vi "Begin.vi"(11 "Image Size":T1=enum."160x120") -> (0 "error out":errorcluster)   [LabVIEW 2012]
doc: "Called before other user functions, this VI is expected to open initial I/O refnums, load in file data, and do all program initialization. Notice that the <B>error out</B> terminal is simply used for data flow. Wiring it to other structures or subVIs ensures that this VI runs first."
uses:
  <vilib>/Rock Robotics/WPI/Camera/WPI_CameraImageSize.ctl
  <vilib>/Rock Robotics/WPI/Camera/WPI_CameraWhite Balance Values.ctl
  <vilib>/Rock Robotics/WPI/Camera/WPI_CameraExposure Values.ctl
  <vilib>/Rock Robotics/WPI/Camera/WPI_CameraFrameRate.ctl
  <vilib>/Rock Robotics/WPI/DriverStation/WPI_DriverStationRobotMode2.ctl
  <vilib>/Rock Robotics/SystemInterfaces/DIO/FPGA_DIOChannel.ctl
  <vilib>/Rock Robotics/SystemInterfaces/AI/FPGA_AIGyroChannel.ctl
  <vilib>/Rock Robotics/WPI/Relay/WPI_RelayDirection.ctl
  <vilib>/Rock Robotics/SystemInterfaces/DIO/FPGA_DIORelayChannel.ctl
  <vilib>/Rock Robotics/SystemInterfaces/AI/FPGA_AIChannel.ctl
  <vilib>/Rock Robotics/SystemInterfaces/DIO/FPGA_DIOPWMChannel.ctl
  <vilib>/Rock Robotics/WPI/Joystick/WPI_JoystickDeviceEnum.ctl
  <vilib>/Rock Robotics/SystemInterfaces/Typedef/FPGA_TypedefDigitalModule.ctl
  Robot Global Data.vi
  <vilib>/Rock Robotics/WPI/MotorControl/WPI_MotorControlOpen Victor.vi
  <vilib>/Rock Robotics/WPI/MotorControl/WPI_MotorControlOpen Jaguar.vi
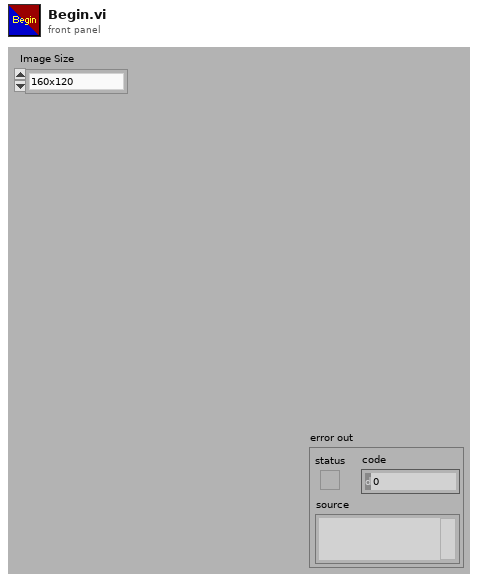
[diagram p1: front panel]
types:
  T1 = typedef "WPI_CameraImageSize.ctl" = enum16{"640x480", "320x240", "160x120"}
  T2 = typedef "FPGA_DIOChannel.ctl" = enum8{"DIO 1", "DIO 2", "DIO 3", "DIO 4", "DIO 5", "DIO 6", "DIO 7", "DIO 8", "DIO 9", "DIO 10", "DIO 11", "DIO 12", "DIO 13", "DIO 14", "Invalid"}
  T3 = typedef "FPGA_TypedefDigitalModule.ctl" = enum16{"Digital Module 1", "Digital Module 2"}
  T4 = typedef "WPI_JoystickDeviceEnum.ctl" = enum16{"USB 1", "USB 2", "USB 3", "USB 4", "Kinect 1", "Kinect 2"}
  T5 = typedef "FPGA_DIOPWMChannel.ctl" = enum8{"PWM 1", "PWM 2", "PWM 3", "PWM 4", "PWM 5", "PWM 6", "PWM 7", "PWM 8", "PWM 9", "PWM 10", "Invalid"}
  T6 = typedef "FPGA_AIChannel.ctl" = enum8{"AI 1", "AI 2", "AI 3", "AI 4", "AI 5", "AI 6", "AI 7", "AI 8", "Invalid"}
  T7 = typedef "FPGA_DIORelayChannel.ctl" = enum8{"Relay 1", "Relay 2", "Relay 3", "Relay 4", "Relay 5", "Relay 6", "Relay 7", "Relay 8", "Invalid"}
  T8 = typedef "WPI_RelayDirection.ctl" = enum16{"Both directions", "Forward only", "Reverse only"}
  T9 = typedef "FPGA_AIGyroChannel.ctl" = enum8{"AI 1", "AI 2", "Invalid"}
  T10 = typedef "WPI_DriverStationRobotMode2.ctl" = enum16{"Autonomous Disabled", "Autonomous Enabled", "Teleop Disabled", "Teleop Enabled", "Timeout", "Finish", "Test Disabled", "Test Enabled"}
  T11 = typedef "WPI_CameraFrameRate.ctl" = u32
  T12 = typedef "WPI_CameraExposure Values.ctl" = enum16{"Auto", "Flicker-free 50 Hz", "Flicker-free 60 Hz", "Hold current"}
  T13 = typedef "WPI_CameraWhite Balance Values.ctl" = enum16{"Auto", "Fixed indoor", "Fixed outdoor 1", "Fixed outdoor 2", "Fixed fluorescent 1", "Fixed fluorescent 2", "Hold current"}
  T14 = typedef "WPI_DigitalInputDevRef.ctl" = cluster{"DevStatus":errorcluster, "DIO Channel":T2, "Digital Module":T3}
  T15 = typedef "WPI_MotorControlDeviceRef.ctl" = cluster{"DeviceStatus":errorcluster, "Type":enum16{"PWM", "CAN"}, "PWM":cluster{"Digital Module":T3, "PWM Channel":T5, "DeadBand":T16}, "CAN":cluster{"Device Number":u8, "Control Mode":T17, "Semaphore":T18, "Max Vout":dbl}, "Invert":bool, "TransformRef":T19, "InvTransformRef":T19}
  T16 = typedef "WPI_PWMDeadband.ctl" = cluster{"Name":string, "maxPositivePwm":i32, "minPositivePwm":i32, "centerPwm":i32, "maxNegativePwm":i32, "minNegativePwm":i32, "angularRange":u16}
  T17 = typedef "WPI_CANJaguar_ControlMode.ctl" = enum8{"Percent VBus", "Current", "Speed", "Position", "Voltage"}
  T18 = typedef "Semaphore RefNum" = refnum<k1>
  T19 = typedef "WPI_PWMTransform_ConPane.ctl" = refnum<vi>
  T20 = typedef "WPI_ServoDeviceRef.ctl" = cluster{"DeviceStatus":errorcluster, "Digital Module":T3, "PWM Channel":T5, "DeadBand":T16}
  T21 = typedef "WPI_RelayDevRef.ctl" = cluster{"DevStatus":errorcluster, "Relay Channel":T7, "Digital Module":T3, "Relay Direction":T8}
  T22 = typedef "WPI_AnalogChannelDevRef.ctl" = cluster{"DevStatus":errorcluster, "Analog Module":T23, "Analog Channel":T6}
  T23 = typedef "FPGA_TypedefAnalogModule.ctl" = enum16{"Analog Module 1", "Analog Module 2"}
  T24 = typedef "WPI_CameraDevRef.ctl" = cluster{"Camera Address":string, "CameraStatus":errorcluster, "Acquire Image Notifier":refnum<notifier>}
  T25 = typedef "WPI_JoystickDevRef.ctl" = cluster{"Device":T4}
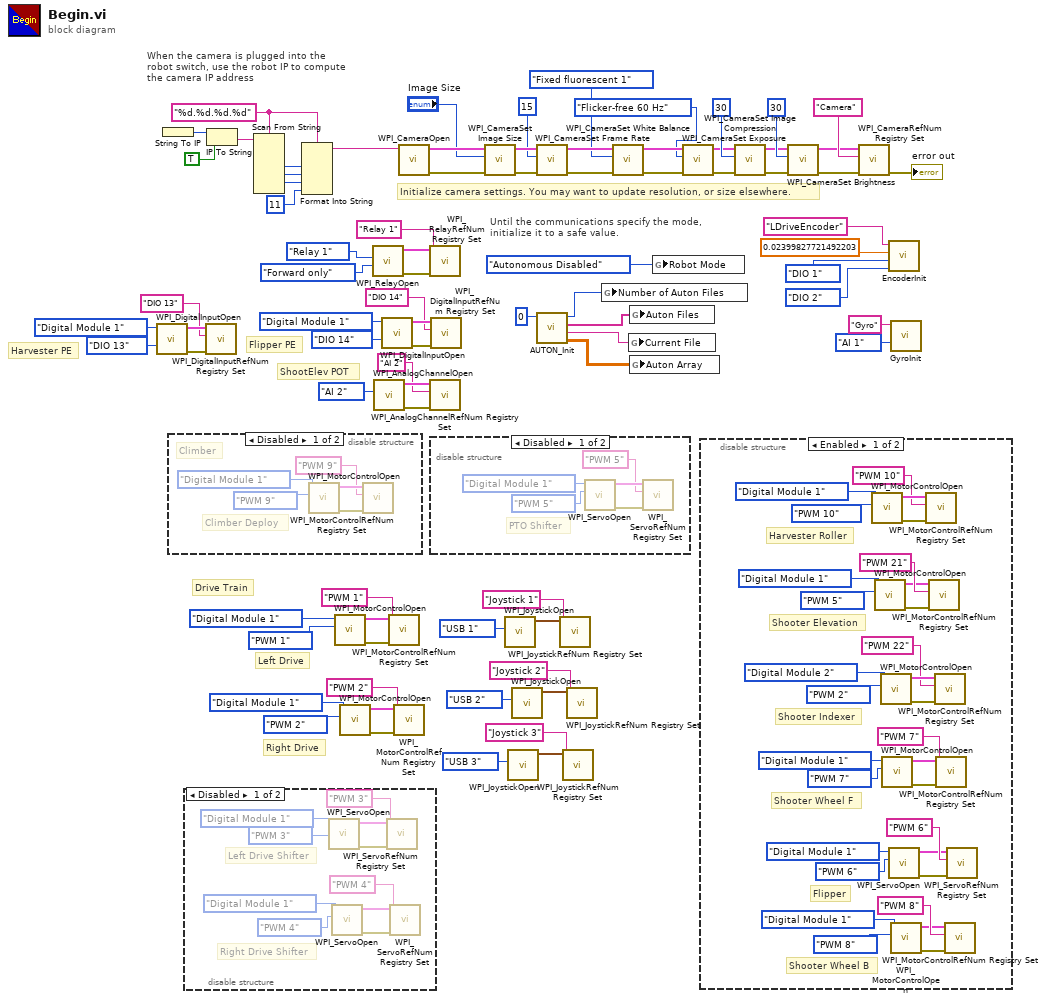
[diagram p0: block diagram]
diagram:
  w53 = "%d.%d.%d.%d" ("format string")
  # "Harvester PE"
  # "Drive Train"
  # "Right Drive"
  # "Left Drive"
  # "ShootElev POT"
  # "Flipper PE"
  # "Until the communications specify the mode,\ninitialize it to a safe value."
  # "When the camera is plugged into the\nrobot switch, use the robot IP to compute\nthe camera IP address"
  # "Initialize camera settings. You may want to update resolution, or size elsewhere."
  n1 = call <vilib>:"WPI_DigitalInputOpen.vi"("DIO Channel"=FPGA_DIOChannel."DIO 13", "Digital Module (Module 1)"=FPGA_TypedefDigitalModule."Digital Module 1") -> ("error out"=w2:errorcluster, "DigitalInputDevRef"=w3:T14)  [unwired: 8 in]
  n2 = String To IP() -> (0:w60:u32)  [unwired: 1 in]
  n3 = disable-structure shown="Disabled" {
    frame Disabled {
      # "Climber Deploy"
      # "Climber"
      n4 = call-poly <vilib>:"WPI_MotorControlOpen.vi"("PWM Channel"=FPGA_DIOPWMChannel."PWM 9", "Digital Module (Module 1)"=FPGA_TypedefDigitalModule."Digital Module 1") -> ("error out"=w83:errorcluster, "MotorControlDeviceRef"=w84:T15)  [unwired: 8 in]
      n5 = call <vilib>:"WPI_MotorControlRefNum Registry Set.vi"("error in (no error)"=w83, "refnum name"="PWM 9", "MotorControlDevRef"=w84) -> ()  [unwired: 7 in, 2 out]
    }
    frame Enabled {
    }
  }
  n6 = disable-structure shown="Disabled" {
    frame Disabled {
      # "Right Drive Shifter"
      # "Left Drive Shifter"
      n7 = call <vilib>:"WPI_ServoOpen.vi"("PWM Channel"=FPGA_DIOPWMChannel."PWM 3", "Digital Module (Module 1)"=FPGA_TypedefDigitalModule."Digital Module 1") -> ("error out"=w88:errorcluster, "ServoDeviceRef"=w89:T20)  [unwired: 8 in]
      n8 = call <vilib>:"WPI_ServoOpen.vi"("PWM Channel"=FPGA_DIOPWMChannel."PWM 4", "Digital Module (Module 1)"=FPGA_TypedefDigitalModule."Digital Module 1") -> ("error out"=w87:errorcluster, "ServoDeviceRef"=w94:T20)  [unwired: 8 in]
      n9 = call <vilib>:"WPI_ServoRefNum Registry Set.vi"("error in (no error)"=w88, "refnum name"="PWM 3", "ServoDeviceRef"=w89) -> ()  [unwired: 7 in, 2 out]
      n10 = call <vilib>:"WPI_ServoRefNum Registry Set.vi"("error in (no error)"=w87, "refnum name"="PWM 4", "ServoDeviceRef"=w94) -> ()  [unwired: 7 in, 2 out]
    }
    frame Enabled {
    }
  }
  n11 = call <vilib>:"WPI_DigitalInputRefNum Registry Set.vi"("error in (no error)"=w2, "refnum name"="DIO 13", "DigitalInputDevRef"=w3) -> ()  [unwired: 7 in, 2 out]
  n12 = IP To String(1:TRUE ("dot notation? (F)"), 2:w60) -> (0:w58:string)
  n13 = Scan From String(format string=w53, input string=w58) -> (output 1=w57:i32, output 2=w56:i32, output 3=w55:i32)  [unwired: 7 in, 3 out]
  n14 = Format Into String(format string=w53, w57, w56, w55, 11 ("Compression")) -> (resulting string=w51:string)  [unwired: 2 in, 1 out]
  n15 = call-poly <vilib>:"WPI_MotorControlOpen.vi"("PWM Channel"=FPGA_DIOPWMChannel."PWM 1", "Digital Module (Module 1)"=FPGA_TypedefDigitalModule."Digital Module 1") -> ("error out"=w15:errorcluster, "MotorControlDeviceRef"=w16:T15)  [unwired: 8 in]
  n16 = call-poly <vilib>:"WPI_MotorControlOpen.vi"("PWM Channel"=FPGA_DIOPWMChannel."PWM 2", "Digital Module (Module 1)"=FPGA_TypedefDigitalModule."Digital Module 1") -> ("error out"=w22:errorcluster, "MotorControlDeviceRef"=w21:T15)  [unwired: 8 in]
  n17 = call <vilib>:"WPI_RelayOpen.vi"("Relay Direction"=WPI_RelayDirection."Forward only", "Relay Channel"=FPGA_DIORelayChannel."Relay 1") -> ("error out"=w38:errorcluster, "RelayDevRef"=w37:T21)  [unwired: 8 in]
  n18 = call <vilib>:"WPI_AnalogChannelOpen.vi"("Analog Channel"=FPGA_AIChannel."AI 2") -> ("error out"=w28:errorcluster, "AIDeviceRef"=w27:T22)  [unwired: 9 in]
  n19 = call <vilib>:"WPI_DigitalInputOpen.vi"("DIO Channel"=FPGA_DIOChannel."DIO 14", "Digital Module (Module 1)"=FPGA_TypedefDigitalModule."Digital Module 1") -> ("error out"=w33:errorcluster, "DigitalInputDevRef"=w32:T14)  [unwired: 8 in]
  n20 = call <vilib>:"WPI_MotorControlRefNum Registry Set.vi"("error in (no error)"=w15, "refnum name"="PWM 1", "MotorControlDevRef"=w16) -> ()  [unwired: 7 in, 2 out]
  n21 = call <vilib>:"WPI_MotorControlRefNum Registry Set.vi"("error in (no error)"=w22, "refnum name"="PWM 2", "MotorControlDevRef"=w21) -> ()  [unwired: 7 in, 2 out]
  n22 = call <vilib>:"WPI_CameraOpen.vi"("Camera Address"=w51) -> ("error out"=w72:errorcluster, "CameraDevRef"=w73:T24)  [unwired: 1 in, 8 out]
  n23 = call <vilib>:"WPI_RelayRefNum Registry Set.vi"("error in (no error)"=w38, "refnum name"="Relay 1", "RelayDevRef"=w37) -> ()  [unwired: 7 in, 2 out]
  n24 = call <vilib>:"WPI_AnalogChannelRefNum Registry Set.vi"("error in (no error)"=w28, "refnum name"="AI 2", "AIDeviceRef"=w27) -> ()  [unwired: 7 in, 2 out]
  n25 = call <vilib>:"WPI_DigitalInputRefNum Registry Set.vi"("error in (no error)"=w33, "refnum name"="DIO 14", "DigitalInputDevRef"=w32) -> ()  [unwired: 7 in, 2 out]
  n26 = disable-structure shown="Disabled" {
    frame Disabled {
      # "PTO Shifter"
      n27 = call <vilib>:"WPI_ServoOpen.vi"("PWM Channel"=FPGA_DIOPWMChannel."PWM 5", "Digital Module (Module 1)"=FPGA_TypedefDigitalModule."Digital Module 1") -> ("error out"=w101:errorcluster, "ServoDeviceRef"=w100:T20)  [unwired: 8 in]
      n28 = call <vilib>:"WPI_ServoRefNum Registry Set.vi"("error in (no error)"=w101, "refnum name"="PWM 5", "ServoDeviceRef"=w100) -> ()  [unwired: 7 in, 2 out]
    }
    frame Enabled {
    }
  }
  n29 = call <vilib>:"WPI_CameraSet Image Size.vi"("error in (no error)"=w72, "Image Size"="Image Size", "CameraDevRef"=w73) -> ("error out"=w71:errorcluster, "CameraDevRef Out"=w74:T24)  [unwired: 7 out]
  n30 = call <vilib>:"WPI_JoystickOpen.vi"("JoystickDevice"=WPI_JoystickDeviceEnum."USB 1") -> ("JoystickDevRef"=w6:T25)  [unwired: 10 in]
  n31 = call <vilib>:"WPI_JoystickOpen.vi"("JoystickDevice"=WPI_JoystickDeviceEnum."USB 3") -> ("JoystickDevRef"=w12:T25)  [unwired: 10 in]
  n32 = call <vilib>:"WPI_JoystickOpen.vi"("JoystickDevice"=WPI_JoystickDeviceEnum."USB 2") -> ("JoystickDevRef"=w11:T25)  [unwired: 10 in]
  n33 = call <vilib>:"WPI_CameraSet Frame Rate.vi"("error in (no error)"=w71, "Frame Rate (fps)"=T11 15, "CameraDevRef"=w74) -> ("error out"=w70:errorcluster, "CameraDevRef Out"=w76:T24)  [unwired: 7 out]
  n34 = call "AUTON_Init.vi"("Default File"=0) -> ("Auton Array"=w45:dbl[][], "Current File"=w46:string, "Auton Files"=w47:string[], "Number of Auton Files"=w48:i64)  [unwired: 7 in]
  n35 = call <vilib>:"WPI_JoystickRefNum Registry Set.vi"("refnum name"="Joystick 1", "JoystickDevRef"=w6) -> ()  [unwired: 8 in, 2 out]
  n36 = call <vilib>:"WPI_JoystickRefNum Registry Set.vi"("refnum name"="Joystick 3", "JoystickDevRef"=w12) -> ()  [unwired: 8 in, 2 out]
  n37 = call <vilib>:"WPI_JoystickRefNum Registry Set.vi"("refnum name"="Joystick 2", "JoystickDevRef"=w11) -> ()  [unwired: 8 in, 2 out]
  n38 = global write "Robot Global Data.vi" "Number of Auton Files"(w48) -> ()
  n39 = call <vilib>:"WPI_CameraSet White Balance.vi"("error in (no error)"=w70, "White Balance"=WPI_CameraWhite_Balance_Values."Fixed fluorescent 1", "CameraDevRef"=w76) -> ("error out"=w69:errorcluster, "CameraDevRef Out"=w75:T24)  [unwired: 7 out]
  n40 = global write "Robot Global Data.vi" "Current File"(w46) -> ()
  n41 = global write "Robot Global Data.vi" "Auton Files"(w47) -> ()
  n42 = global write "Robot Global Data.vi" "Auton Array"(w45) -> ()
  n43 = global write "Robot Global Data.vi" "Robot Mode"(WPI_DriverStationRobotMode2."Autonomous Disabled" ("Robot Mode")) -> ()
  n44 = call <vilib>:"WPI_CameraSet Exposure.vi"("error in (no error)"=w69, "Exposure"=WPI_CameraExposure_Values."Flicker-free 60 Hz", "CameraDevRef"=w75) -> ("error out"=w68:errorcluster, "CameraDevRef Out"=w78:T24)  [unwired: 7 out]
  n45 = disable-structure shown="Enabled" {
    frame Enabled {
      # "Shooter Wheel B"
      # "Flipper"
      # "Shooter Indexer"
      # "Shooter Elevation"
      # "Harvester Roller"
      # "Shooter Wheel F"
      n46 = call-poly <vilib>:"WPI_MotorControlOpen.vi"("PWM Channel"=FPGA_DIOPWMChannel."PWM 10", "Digital Module (Module 1)"=FPGA_TypedefDigitalModule."Digital Module 1") -> ("error out"=w125:errorcluster, "MotorControlDeviceRef"=w126:T15)  [unwired: 8 in]
      n47 = call-poly <vilib>:"WPI_MotorControlOpen.vi"("PWM Channel"=FPGA_DIOPWMChannel."PWM 5", "Digital Module (Module 1)"=FPGA_TypedefDigitalModule."Digital Module 1") -> ("error out"=w119:errorcluster, "MotorControlDeviceRef"=w118:T15)  [unwired: 8 in]
      n48 = call-poly <vilib>:"WPI_MotorControlOpen.vi"("PWM Channel"=FPGA_DIOPWMChannel."PWM 2", "Digital Module (Module 1)"=FPGA_TypedefDigitalModule."Digital Module 2") -> ("error out"=w114:errorcluster, "MotorControlDeviceRef"=w115:T15)  [unwired: 8 in]
      n49 = call-poly <vilib>:"WPI_MotorControlOpen.vi"("PWM Channel"=FPGA_DIOPWMChannel."PWM 7", "Digital Module (Module 1)"=FPGA_TypedefDigitalModule."Digital Module 1") -> ("error out"=w128:errorcluster, "MotorControlDeviceRef"=w129:T15)  [unwired: 8 in]
      n50 = call <vilib>:"WPI_ServoOpen.vi"("PWM Channel"=FPGA_DIOPWMChannel."PWM 6", "Digital Module (Module 1)"=FPGA_TypedefDigitalModule."Digital Module 1") -> ("error out"=w107:errorcluster, "ServoDeviceRef"=w108:T20)  [unwired: 8 in]
      n51 = call-poly <vilib>:"WPI_MotorControlOpen.vi"("PWM Channel"=FPGA_DIOPWMChannel."PWM 8", "Digital Module (Module 1)"=FPGA_TypedefDigitalModule."Digital Module 1") -> ("error out"=w104:errorcluster, "MotorControlDeviceRef"=w103:T15)  [unwired: 8 in]
      n52 = call <vilib>:"WPI_MotorControlRefNum Registry Set.vi"("error in (no error)"=w125, "refnum name"="PWM 10", "MotorControlDevRef"=w126) -> ()  [unwired: 7 in, 2 out]
      n53 = call <vilib>:"WPI_MotorControlRefNum Registry Set.vi"("error in (no error)"=w119, "refnum name"="PWM 21", "MotorControlDevRef"=w118) -> ()  [unwired: 7 in, 2 out]
      n54 = call <vilib>:"WPI_MotorControlRefNum Registry Set.vi"("error in (no error)"=w114, "refnum name"="PWM 22", "MotorControlDevRef"=w115) -> ()  [unwired: 7 in, 2 out]
      n55 = call <vilib>:"WPI_MotorControlRefNum Registry Set.vi"("error in (no error)"=w128, "refnum name"="PWM 7", "MotorControlDevRef"=w129) -> ()  [unwired: 7 in, 2 out]
      n56 = call <vilib>:"WPI_MotorControlRefNum Registry Set.vi"("error in (no error)"=w104, "refnum name"="PWM 8", "MotorControlDevRef"=w103) -> ()  [unwired: 7 in, 2 out]
      n57 = call <vilib>:"WPI_ServoRefNum Registry Set.vi"("error in (no error)"=w107, "refnum name"="PWM 6", "ServoDeviceRef"=w108) -> ()  [unwired: 7 in, 2 out]
    }
    frame Disabled {
    }
  }
  n58 = call <vilib>:"WPI_CameraSet Image Compression.vi"("error in (no error)"=w68, "Compression"=30, "CameraDevRef"=w78) -> ("error out"=w67:errorcluster, "CameraDevRef Out"=w77:T24)  [unwired: 7 out]
  n59 = call <vilib>:"WPI_CameraSet Brightness.vi"("error in (no error)"=w67, "Brightness"=30, "CameraDevRef"=w77) -> ("error out"=w65:errorcluster, "CameraDevRef Out"=w66:T24)  [unwired: 7 out]
  n60 = call <vilib>:"WPI_CameraRefNum Registry Set.vi"("error in (no error)"=w65, "refnum name"="Camera", "CameraDevRef"=w66) -> ("error out"=→"error out":errorcluster)  [unwired: 8 out]
  n61 = call "EncoderInit.vi"("refnum name"="LDriveEncoder", "DistancePerCount"=0.02399827721492203, "DIO Channel"=FPGA_DIOChannel."DIO 1", "DIO Channel 2"=FPGA_DIOChannel."DIO 2") -> ()  [unwired: 7 in]
  n62 = call "GyroInit.vi"("refnum name"="Gyro", "Analog Channel"=FPGA_AIGyroChannel."AI 1") -> ()  [unwired: 8 in]
